vi "LCC Read Actual Value.vi"(8 "error in (no error)":errorcluster caption="Fehler (Eingang, kein Fehler)", 11 "Channel Handle":i64) -> (0 "error out":errorcluster caption="Fehler (Ausgang)", 3 "Actual Value":dbl)   [LabVIEW 2021, in "labbCAN_Controller_API.lvlib"]
doc: "LCC_Func long LCC_CALL LCC_ReadActualValue(dev_hdl ChanHdl, double *pfActualValue);"
uses:
  labbCAN_Controller_API.lvlib
  labbCAN_Controller_API.dll
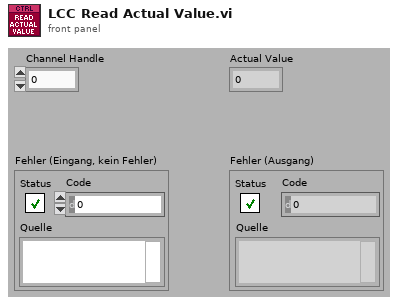
[diagram p1: front panel]
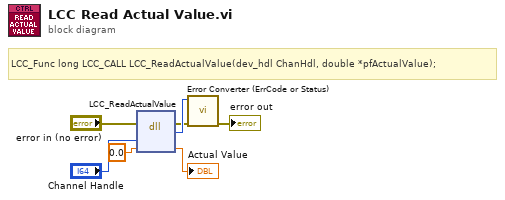
[diagram p0: block diagram]
diagram:
  # "LCC_Func long LCC_CALL LCC_ReadActualValue(dev_hdl ChanHdl, double *pfActualValue);"
  n1 = dll-call lib="C:/Users/olaja/AppData/Local/CETONI_SDK/labbCAN_Controller_API.*" fn="LCC_ReadActualValue"(error in="error in (no error)", "ChanHdl"="Channel Handle", "pfActualValue"=0.0) -> (error out=w2:errorcluster, "Rückgabetyp"=w3:i32, "pfActualValue"=→"Actual Value":dbl)  [unwired: 3 in, 1 out]
  n2 = call "Error Converter (ErrCode or Status).vi"("error in (no error)"=w2, "error code"=w3) -> ("error out"=→"error out":errorcluster)  [unwired: 9 in]
